vi "LVDemo1-Z.vi"() -> ()   [LabVIEW 2016]
uses:
  toupcam.dll
  toupcam_labview.dll
panel:
  out "x/y":dbl
  out "10^x":dbl
  out "连接的字符串":string
  out "路径":path
  in  "下降步长":i32=3
  in  "step":i64(ring) items=["1", "10", "100", "1000", "10000"]
  in  "停止":bool
  in  "开始拍图":bool
  in  "Temp 3":i32
  in  "Tint 3":i32
  in  "Expotime 3":u32
  in  "ExpoGain 3":u16
  in  "Still_Width 2":i32
  in  "Still_Height 2":i32
  in  "Tab":T1(tab)
  in  "Color Default":bool
  in  "Brightness":i32(slide) scale=-64.0..64.0
  in  "Contrast":i32(slide) scale=-100.0..100.0
  in  "Gamma":i32(slide) scale=20.0..180.0
  in  "Hue":i32(slide) scale=-180.0..180.0
  in  "Saturation":i32(slide) scale=0.0..255.0
  in  "AutoExpo":bool
  in  "ExpoDefault":bool
  in  "Expotime":u32(slide) scale=100.0..3600000000.0
  in  "ExpoGain":u16(slide) scale=100.0..5000.0
  in  "AutoWB":bool
  in  "WBDefault":bool
  in  "Tint":i32(slide) scale=200.0..2500.0
  in  "Temp":i32(slide) scale=2000.0..15000.0
  in  "Bin/Skip Mode":bool
  in  "Chrome/Mono":bool
  in  "HFlip":bool
  in  "VFlip":bool
  in  "Frame Speed":u8(slide) scale=0.0..2.0
  out "Video":T2(plugin-control)
  in  "Cap Still Image":bool
  in  "Still Image Resolution":u16(ring) items=["3840*2160", "1920*1080"]
  in  "Cap Live Image":bool
  in  "Stop":bool
  in  "Live Resolution":u16(ring) items=["3840*2160", "1920*1080"]
  in  "?":enum32{"选项卡 1"}(tab)
  in  "Expotime_def":u32
  in  "ExpoGain_def":u16
  in  "ExpoGain_Max":u16
  in  "ExpoGain_Min":u16
  in  "Height":i32
  in  "Width":i32
  in  "Expotime_Max":u32
  in  "Expotime_Min":u32
  in  "speed":u8
  in  "height2":i32
  in  "width2":i32
  in  "Mode":bool
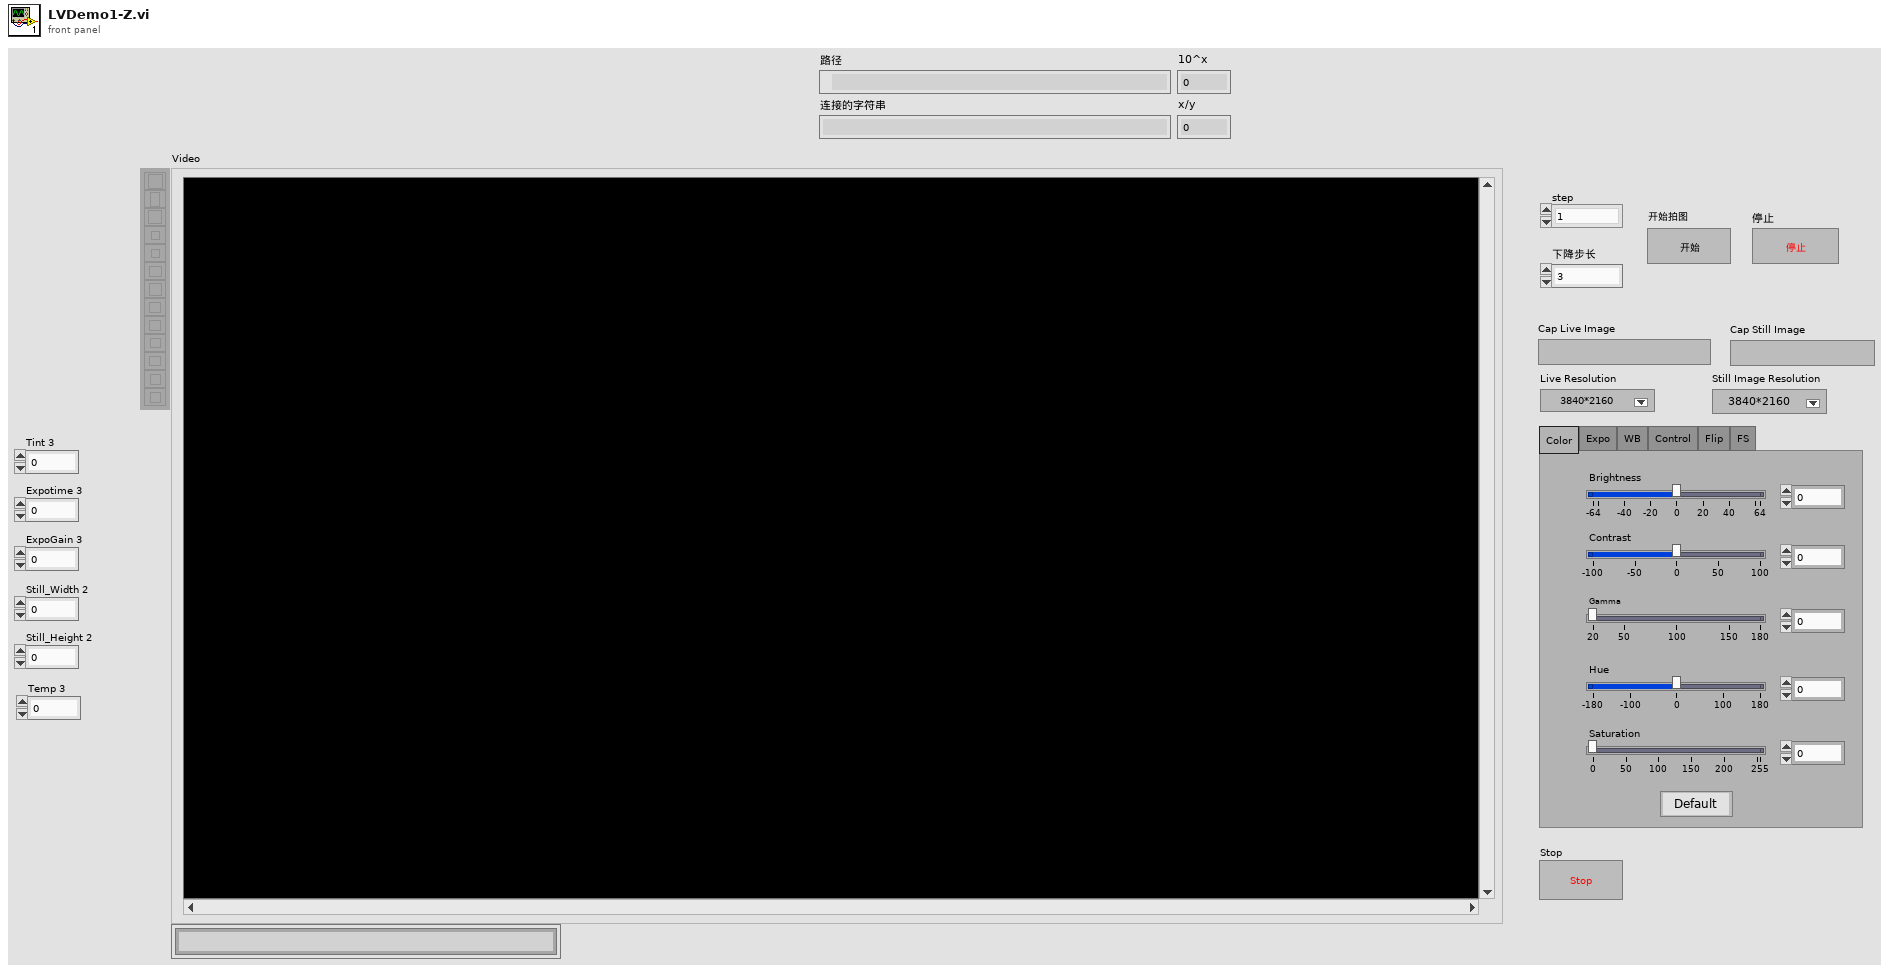
[diagram p1: front panel]
types:
  T1 = enum32{"Color", "Expo", "WB", "Control", "Flip", "FS"}
  T2 = typedef "IMAQ Image.ctl" = refnum<image>
  T3 = enum8{"Enabled", "Disabled", "Disabled and Grayed Out"}
  T4 = typedef "Image Type" = u32
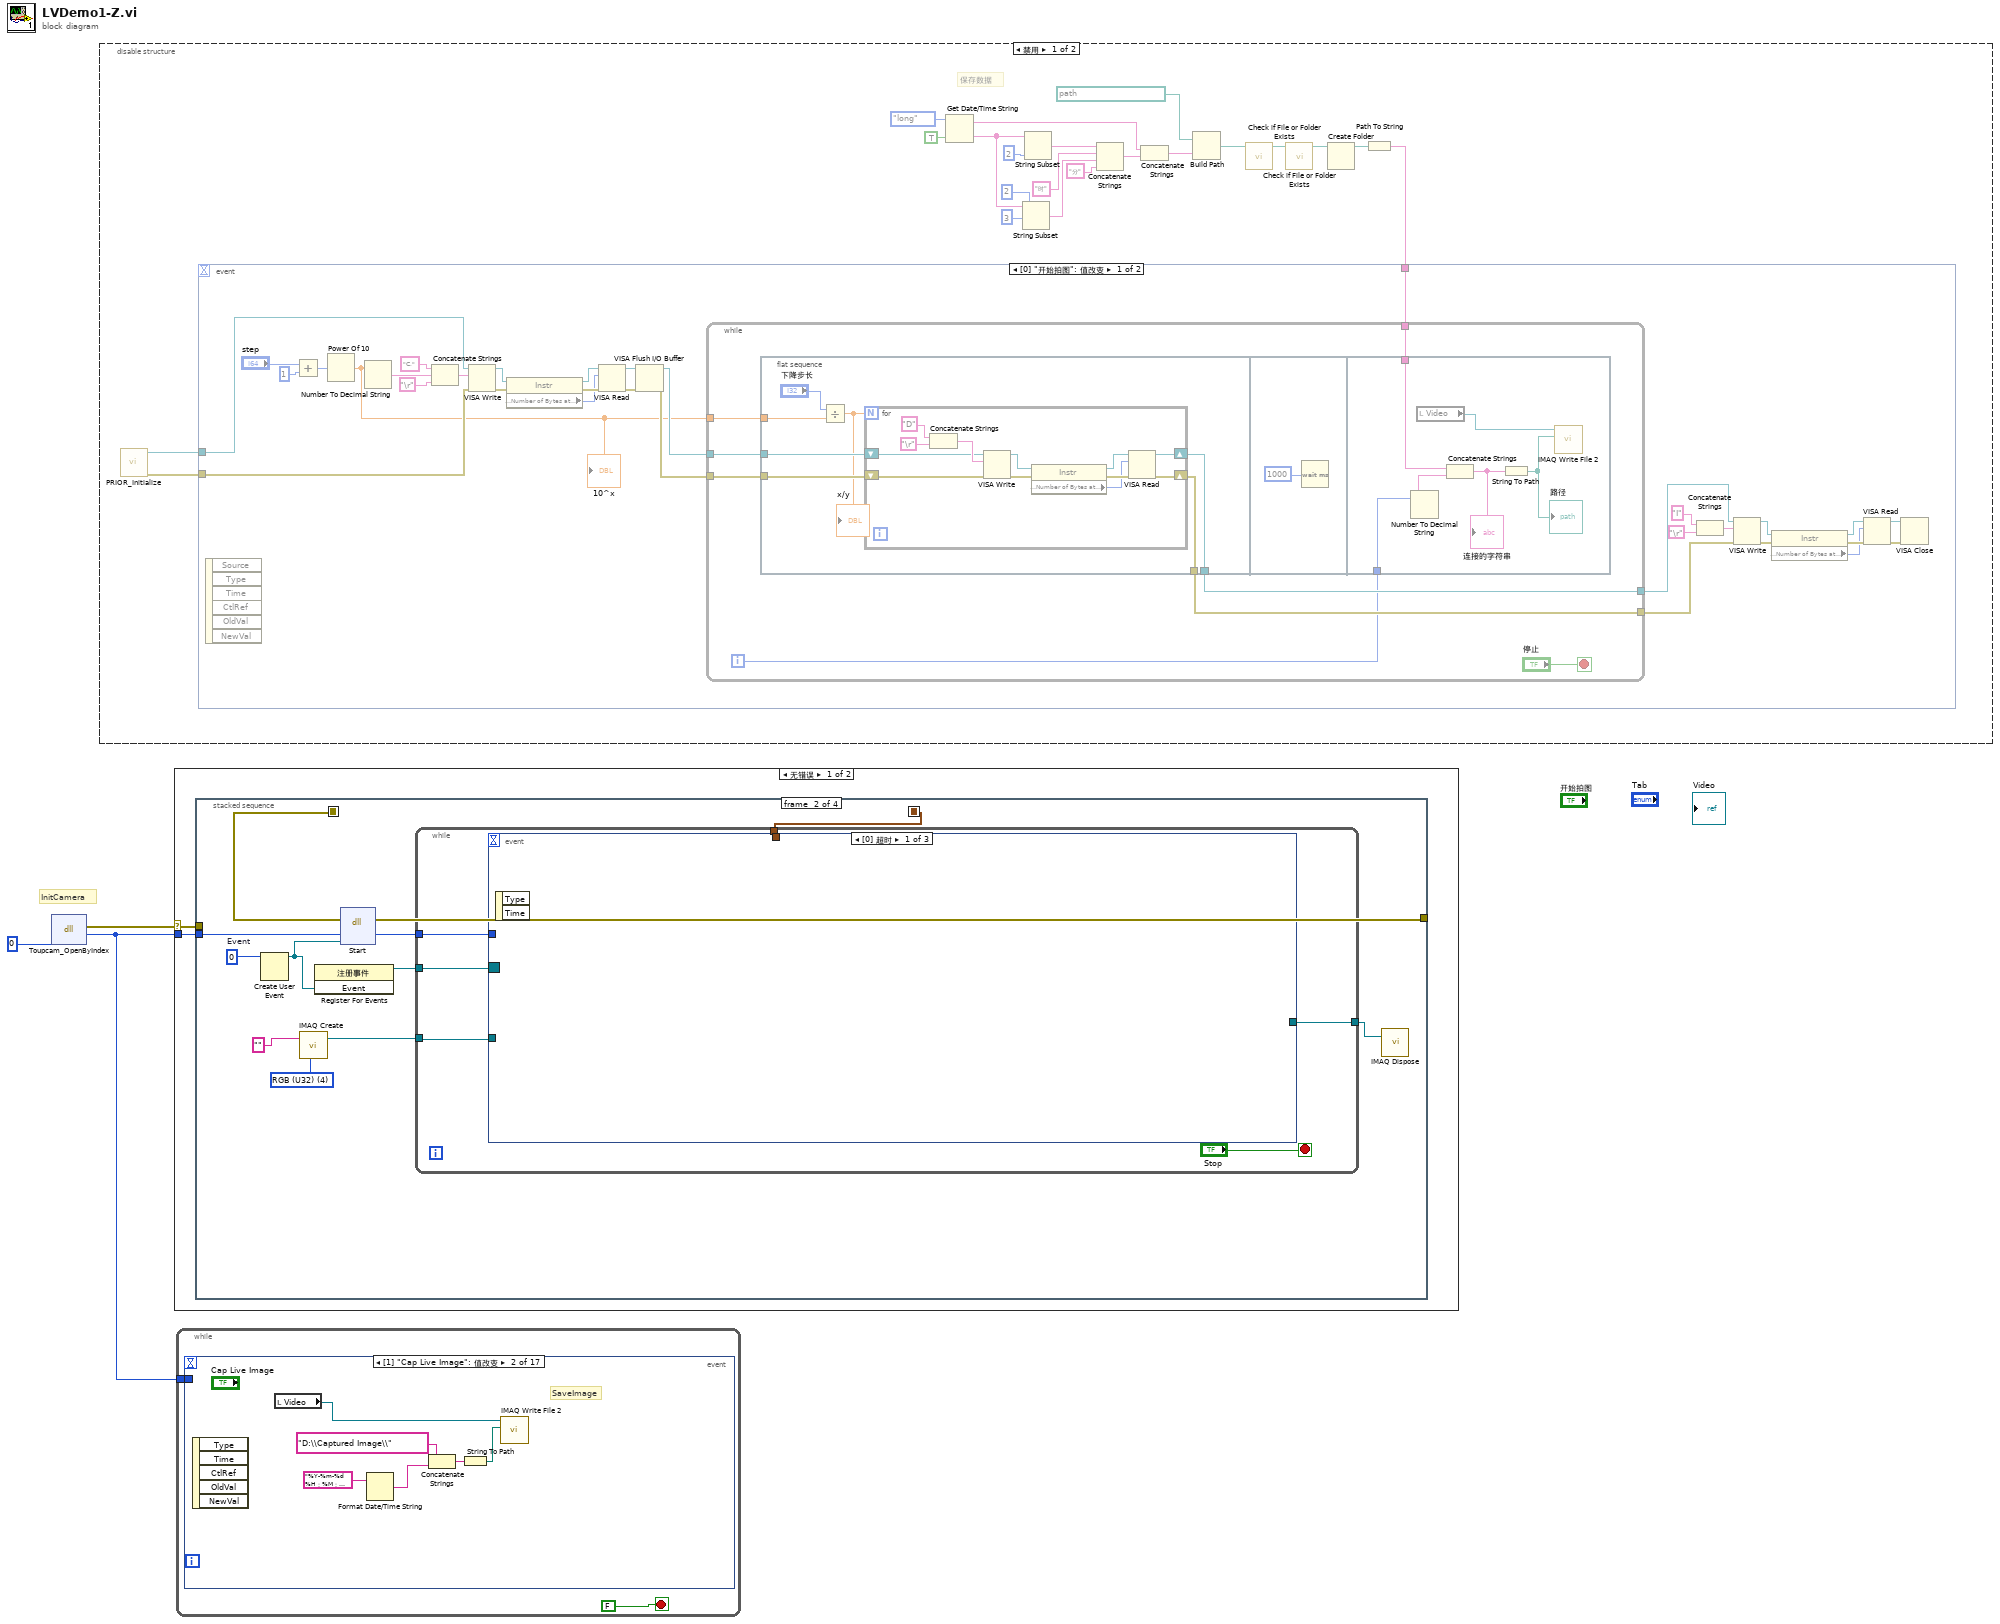
[diagram p0: block diagram]
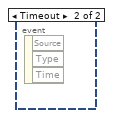
[diagram p2: hidden frame]
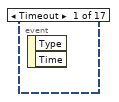
[diagram p4: hidden frame]
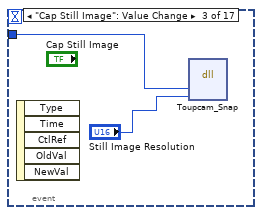
[diagram p5: hidden frame]
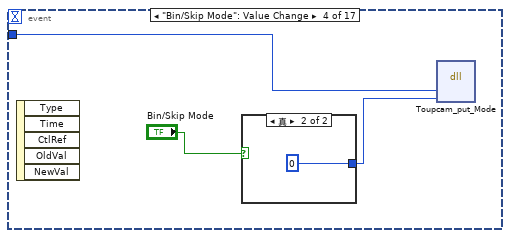
[diagram p6: hidden frame]
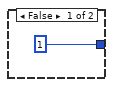
[diagram p7: hidden frame]
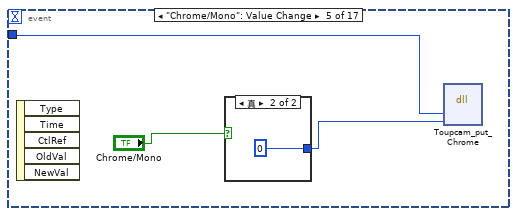
[diagram p8: hidden frame]
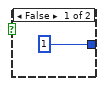
[diagram p9: hidden frame]
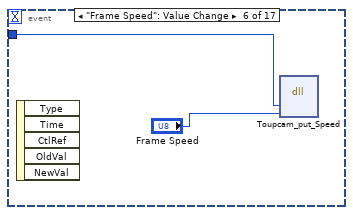
[diagram p10: hidden frame]
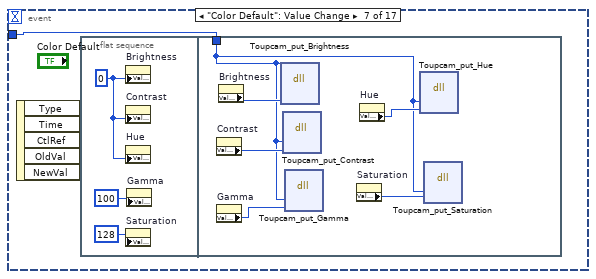
[diagram p11: hidden frame]
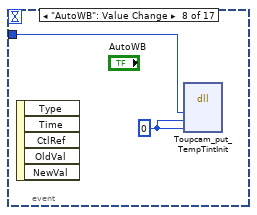
[diagram p12: hidden frame]
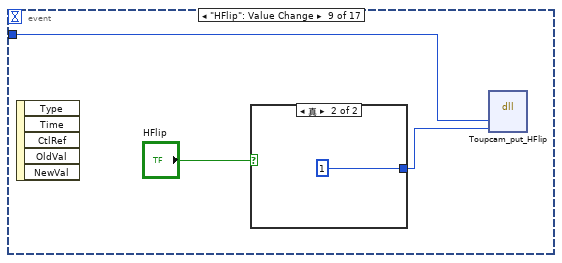
[diagram p13: hidden frame]
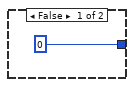
[diagram p14: hidden frame]
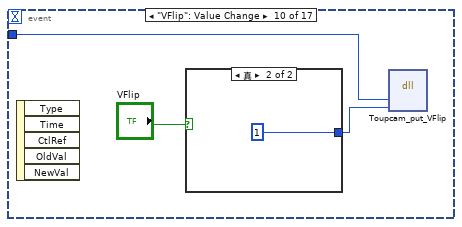
[diagram p15: hidden frame]
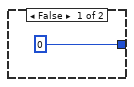
[diagram p16: hidden frame]
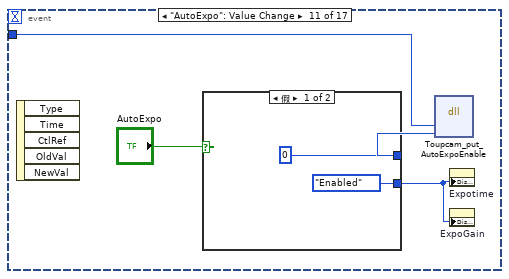
[diagram p17: hidden frame]
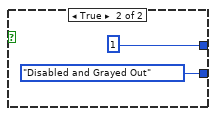
[diagram p18: hidden frame]
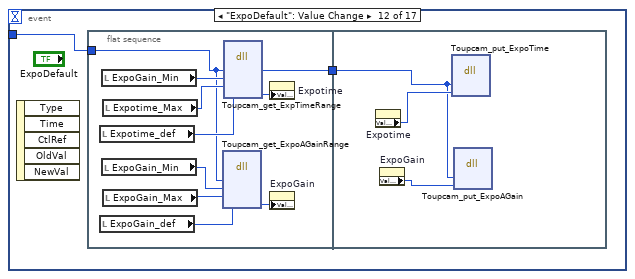
[diagram p19: hidden frame]
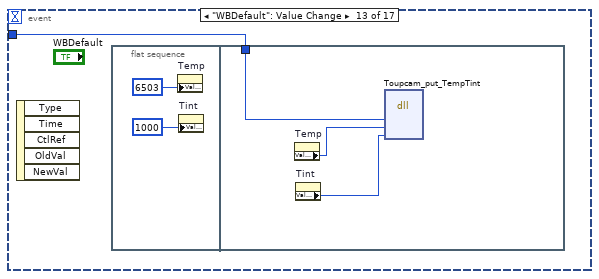
[diagram p20: hidden frame]
diagram:
  # "InitCamera"
  n1 = dll-call lib="PTH2=abs E膜片\t膜片钳程序自动拍图toupcam.dll" fn="Toupcam_OpenByIndex"("Index"=0) -> (error out=w3:errorcluster, "return type"=w2:i32)  [unwired: 4 in, 1 out]
  n2 = disable-structure shown="禁用" {
    frame Disabled {
      # "保存数据"
      n3 = call "PRIOR_Initialize.vi"() -> ("错误输出"=w23:errorcluster, "VISA资源名称输出"=w24:refnum<visa-resource-name>)  [unwired: 10 in]
      n4 = Get Date/Time String(date format (0)=enum16{"short", "long", "abbreviated"}."long" ("日期格式(0)"), want seconds? (F)=TRUE ("需要秒？(F)")) -> (date string=w22:string, time string=w13:string)  [unwired: 1 in]
      n5 = String Subset(string=w13, offset (0)=3 ("偏移量(0)"), length (rest)=2 ("长度（剩余）")) -> (substring=w17:string)
      n6 = String Subset(string=w13, length (rest)=2 ("长度（剩余）")) -> (substring=w19:string)  [unwired: 1 in]
      n7 = Concatenate Strings(w19, "时" ("字符串"), w17, "分" ("字符串")) -> (w18:string)
      n8 = Concatenate Strings(w22, w18) -> (w10:string)
      n9 = Build Path(base path=path "E:/膜片/图片和视频" ("文件路径（使用对话框）"), name or relative path=w10) -> (appended path=w4:path)
      n10 = call <vilib>:"Check if File or Folder Exists.vi"("path"=w4) -> ("dup path"=w6:path)  [unwired: 8 in, 2 out]
      n11 = call <vilib>:"Check if File or Folder Exists.vi"("path"=w6) -> ("dup path"=w5:path)  [unwired: 8 in, 2 out]
      n12 = Create Folder(path (use dialog)=w5) -> (created path=w8:path)  [unwired: 2 in, 2 out]
      n13 = Path To String(path=w8) -> (string=w7:string)
      n14 = event shown="[0] \"开始拍图\": 值改变" {
        selector: _ -> [_ _]
        dyn-events: _ -> [_ _]
        timeout: _ -> [_ _]
        tunnel: w24 -> [w56 _]
        tunnel: w23 -> [w55 _]
        tunnel: w7 -> [w25 _]
        event "开始拍图": Value Change {
          n15 = event-data() -> ()  [unwired: 1 in, 6 out]
          n16 = Add(x="step", y=i64 1) -> (x+y=w43:i64)
          n17 = Power Of 10(x=w43) -> (10^x=w26:dbl)
          "10^x" <- w26
          n18 = Number To Decimal String(number=w26) -> (decimal integer string=w45:string)  [unwired: 1 in]
          n19 = Concatenate Strings("C," ("写入缓冲区"), w45, "\r") -> (w47:string)
          n20 = VISA Write ("VISA写入")(VISA resource name=w56, write buffer=w47, error in (no error)=w55) -> (VISA resource name out=w51:refnum<visa-resource-name>, error out=w52:errorcluster)  [unwired: 1 out]
          n21 = property class="Instr"(reference=w51, error in=w52) -> (reference out=w50:refnum<visa-resource-name>, error out=w49:errorcluster, "Serial Settings:Number of Bytes at Serial Port"=w28:u32)
          n22 = VISA Read(VISA resource name=w50, byte count=w28, error in (no error)=w49) -> (VISA resource name out=w42:refnum<visa-resource-name>, error out=w41:errorcluster)  [unwired: 2 out]
          n23 = VISA Flush I/O Buffer(VISA resource name=w42, error in (no error)=w41) -> (VISA resource name out=w39:refnum<visa-resource-name>, error out=w40:errorcluster)  [unwired: 1 in]
          n24 = while {
            tunnel: [w64] -> w30
            tunnel: [w63] -> w29
            tunnel: w40 -> [w61]
            tunnel: w39 -> [w60]
            tunnel: w26 -> [w58]
            tunnel: w25 -> [w57]
            i -> [w62]
            stop <- "停止" stop-if-true
            n25 = flat-sequence {
              tunnel: [w71] -> w64
              tunnel: [w70] -> w63
              tunnel: w61 -> [w69]
              tunnel: w60 -> [w68]
              tunnel: w58 -> [w66]
              tunnel: w62 -> [w87]
              tunnel: w57 -> [w86]
              frame #0 {
                n26 = Divide(x="下降步长", y=w66) -> (x/y=w65:dbl)
                "x/y" <- w65
                n27 = for {
                  N: w65 -> [_]
                  shift-right: [w76] -> w70
                  shift-left: w69 -> [w75]
                  shift-right: [w77] -> w71
                  shift-left: w68 -> [w72]
                  n28 = Concatenate Strings("D" ("写入缓冲区"), "\r") -> (w83:string)
                  n29 = VISA Write ("VISA写入")(VISA resource name=w72, write buffer=w83, error in (no error)=w75) -> (VISA resource name out=w73:refnum<visa-resource-name>, error out=w78:errorcluster)  [unwired: 1 out]
                  n30 = property class="Instr"(reference=w73, error in=w78) -> (reference out=w79:refnum<visa-resource-name>, error out=w80:errorcluster, "Serial Settings:Number of Bytes at Serial Port"=w74:u32)
                  n31 = VISA Read(VISA resource name=w79, byte count=w74, error in (no error)=w80) -> (VISA resource name out=w77:refnum<visa-resource-name>, error out=w76:errorcluster)  [unwired: 2 out]
                }
              }
              frame #1 {
                n32 = Wait (ms)(milliseconds to wait=u32 1000 ("等待时间（毫秒）")) -> ()  [unwired: 1 out]
              }
              frame #2 {
                n33 = Number To Decimal String(number=w87) -> (decimal integer string=w85:string)  [unwired: 1 in]
                n34 = local read "Video"() -> (w90:T2)
                n35 = Concatenate Strings(w86, w85) -> (w89:string)
                "连接的字符串" <- w89
                n36 = String To Path(string=w89) -> (path=w88:path)
                "路径" <- w88
                n37 = call-poly "IMAQ Write File 2"("File Path"=w88, "Image"=w90) -> ()  [unwired: 8 in, 2 out]
              }
            }
          }
          n38 = Concatenate Strings("I" ("写入缓冲区"), "\r") -> (w31:string)
          n39 = VISA Write ("VISA写入")(VISA resource name=w30, write buffer=w31, error in (no error)=w29) -> (VISA resource name out=w37:refnum<visa-resource-name>, error out=w38:errorcluster)  [unwired: 1 out]
          n40 = property class="Instr"(reference=w37, error in=w38) -> (reference out=w36:refnum<visa-resource-name>, error out=w35:errorcluster, "Serial Settings:Number of Bytes at Serial Port"=w34:u32)
          n41 = VISA Read(VISA resource name=w36, byte count=w34, error in (no error)=w35) -> (VISA resource name out=w53:refnum<visa-resource-name>, error out=w54:errorcluster)  [unwired: 2 out]
          n42 = VISA Close(VISA resource name=w53, error in (no error)=w54) -> ()  [unwired: 1 out]
        }
        event Timeout {
          n43 = event-data() -> ()  [unwired: 1 in, 3 out]
        }
      }
    }
    frame Enabled {
    }
  }
  n44 = case shown="无错误" w3 {
    selector: w3 -> [w91 _]
    tunnel: w2 -> [w92 _]
    frame No Error {
      n45 = stacked-sequence {
        seq-local: [w113 _ _ _] -> [_ w159 _ _]
        seq-local: [w111 _ _ _] -> [_ w158 _ _]
        tunnel: w92 -> [w96 w156 w219 w222]
        tunnel: w91 -> [w111 _ _ w221]
        tunnel: [_ w157 _ _] -> _
        frame #0 {
          w93 = T3."Disabled and Grayed Out" ("禁用")
          w134 = 0
          # "SetSliderRange"
          # "SetCameraResolution"
          # "CameraResolution"
          # "SetSliderDefault"
          n46 = dll-call lib="PTH2=abs E膜片\t膜片钳程序自动拍图toupcam.dll" fn="Toupcam_put_AutoExpoEnable"("htoupcam"=w96, "bAutoExposure"=FALSE) -> ()  [unwired: 6 in, 2 out]
          n47 = dll-call lib="PTH2=abs E膜片\t膜片钳程序自动拍图toupcam.dll" fn="Toupcam_put_ExpoTime"("htoupcam"=w96, "Time"=5000) -> ()  [unwired: 6 in, 2 out]
          n48 = dll-call lib="PTH2=abs E膜片\t膜片钳程序自动拍图toupcam.dll" fn="Toupcam_get_ExpTimeRange"("htoupcam"=w96, "nMin"="Expotime_Min", "nMax"="Expotime_Max", "ndef"="Expotime_def") -> ("nMin"=w116:u32, "nMax"=w115:u32, "ndef"=w114:u32)  [unwired: 5 in, 2 out]
          n49 = dll-call lib="PTH2=abs E膜片\t膜片钳程序自动拍图toupcam.dll" fn="Toupcam_get_ExpoAGainRange"("htoupcam"=w96, "nmin"="ExpoGain_Min", "nmax"="ExpoGain_Max", "ndef"="ExpoGain_def") -> ("nmin"=w125:u16, "nmax"=w124:u16, "ndef"=w123:u16)  [unwired: 5 in, 2 out]
          n50 = property on="Expotime" class="Slide (strict)"("Scale.Minimum"=w116, "Scale.Maximum"=w115, "Value"=w114) -> ()  [unwired: 2 in, 2 out]
          n51 = property on="ExpoGain" class="Slide (严格)"("Scale.Minimum"=w125, "Scale.Maximum"=w124, "Value"=w123) -> ()  [unwired: 2 in, 2 out]
          n52 = dll-call lib="PTH2=abs E膜片\t膜片钳程序自动拍图toupcam.dll" fn="Toupcam_get_ResolutionNumber"("htoupcam"=w96) -> ("返回类型"=w102:u32, "htoupcam"=w101:i32)  [unwired: 3 in, 2 out]
          n53 = dll-call lib="PTH2=abs E膜片\t膜片钳程序自动拍图toupcam.dll" fn="Toupcam_get_Mode"("htoupcam"=w96, "bMode"="Mode") -> ("返回类型"=w95:i32)  [unwired: 5 in, 2 out]
          n54 = property on="Expotime" class="Slide (strict)"("DisabledEnum"=w93) -> ()  [unwired: 2 in, 2 out]
          n55 = property on="ExpoGain" class="Slide (strict)"("DisabledEnum"=w93) -> ()  [unwired: 2 in, 2 out]
          n56 = Equal To 0?(x=w95) -> (x = 0?=w94:bool)
          n57 = dll-call lib="PTH2=abs E膜片\t膜片钳程序自动拍图toupcam.dll" fn="Toupcam_get_MaxSpeed"("htoupcam"=w96) -> ("返回类型"=w106:u8)  [unwired: 4 in, 2 out]
          n58 = dll-call lib="PTH2=abs E膜片\t膜片钳程序自动拍图toupcam.dll" fn="Toupcam_get_Speed"("htoupcam"=w96, "speed"="speed") -> ("htoupcam"=w104:i32, "speed"=w107:u8)  [unwired: 4 in, 2 out]
          n59 = for {
            N: w102 -> [_]
            tunnel: w101 -> [w148]
            tunnel: [w139] -> w100 mode=indexing
            i -> [w140]
            # "Enum Res"
            n60 = dll-call lib="PTH2=abs E膜片\t膜片钳程序自动拍图toupcam.dll" fn="Toupcam_get_Resolution"("htoupcam"=w148, "ResNum"=w140, "pWidth"="width2", "pHeight"="height2") -> ("pWidth"=w142:i32, "pHeight"=w141:i32)  [unwired: 6 in, 2 out]
            n61 = Number To Decimal String(number=w142) -> (decimal integer string=w143:string)  [unwired: 1 in]
            n62 = Number To Decimal String(number=w141) -> (decimal integer string=w145:string)  [unwired: 1 in]
            n63 = Concatenate Strings(w143, "*", w145) -> (w139:string)
          }
          n64 = case shown="假" w94 {
            frame True {
              n65 = property on="Bin/Skip Mode" class="Bool (严格)"("DisabledEnum"=T3."Enabled" ("禁用")) -> ()  [unwired: 2 in, 2 out]
            }
            frame False {
              n66 = property on="Bin/Skip Mode" class="Bool (严格)"("DisabledEnum"=T3."Disabled and Grayed Out" ("禁用")) -> ()  [unwired: 2 in, 2 out]
            }
          }
          n67 = property on="Frame Speed" class="Slide (严格)"("Value"=w107, "Scale.Maximum"=w106, "Scale.Minimum"=0) -> ()  [unwired: 2 in, 2 out]
          n68 = dll-call lib="PTH2=abs E膜片\t膜片钳程序自动拍图toupcam.dll" fn="Toupcam_get_MonoMode"("htoupcam"=w104) -> ("返回类型"=w103:i32)  [unwired: 4 in, 2 out]
          n69 = case shown="0, 默认" w103 {
            frame 0, Default {
              w149 = T3."Disabled and Grayed Out" ("禁用")
              # "Mono"
              n70 = property on="Brightness" class="Slide (严格)"("DisabledEnum"=w149) -> ()  [unwired: 2 in, 2 out]
              n71 = property on="Hue" class="Slide (严格)"("DisabledEnum"=w149) -> ()  [unwired: 2 in, 2 out]
              n72 = property on="Contrast" class="Slide (严格)"("DisabledEnum"=w149) -> ()  [unwired: 2 in, 2 out]
              n73 = property on="Gamma" class="Slide (严格)"("DisabledEnum"=w149) -> ()  [unwired: 2 in, 2 out]
              n74 = property on="AutoWB" class="Bool"("DisabledEnum"=w149) -> ()  [unwired: 2 in, 2 out]
              n75 = property on="Temp" class="Slide (严格)"("DisabledEnum"=w149) -> ()  [unwired: 2 in, 2 out]
              n76 = property on="Tint" class="Slide (严格)"("DisabledEnum"=w149) -> ()  [unwired: 2 in, 2 out]
              n77 = property on="Saturation" class="Slide (严格)"("DisabledEnum"=w149) -> ()  [unwired: 2 in, 2 out]
              n78 = property on="WBDefault" class="Bool"("DisabledEnum"=w149) -> ()  [unwired: 2 in, 2 out]
              n79 = property on="Color Default" class="Bool"("DisabledEnum"=w149) -> ()  [unwired: 2 in, 2 out]
            }
            frame 1 {
              w150 = T3."Enabled" ("禁用")
              # "Mono"
              n80 = property on="Brightness" class="Slide (严格)"("DisabledEnum"=w150) -> ()  [unwired: 2 in, 2 out]
              n81 = property on="Hue" class="Slide (严格)"("DisabledEnum"=w150) -> ()  [unwired: 2 in, 2 out]
              n82 = property on="Contrast" class="Slide (严格)"("DisabledEnum"=w150) -> ()  [unwired: 2 in, 2 out]
              n83 = property on="Gamma" class="Slide (严格)"("DisabledEnum"=w150) -> ()  [unwired: 2 in, 2 out]
              n84 = property on="AutoWB" class="Bool"("DisabledEnum"=w150) -> ()  [unwired: 2 in, 2 out]
              n85 = property on="Temp" class="Slide (严格)"("DisabledEnum"=w150) -> ()  [unwired: 2 in, 2 out]
              n86 = property on="Tint" class="Slide (严格)"("DisabledEnum"=w150) -> ()  [unwired: 2 in, 2 out]
              n87 = property on="Saturation" class="Slide (严格)"("DisabledEnum"=w150) -> ()  [unwired: 2 in, 2 out]
              n88 = property on="WBDefault" class="Bool"("DisabledEnum"=w150) -> ()  [unwired: 2 in, 2 out]
              n89 = property on="Color Default" class="Bool"("DisabledEnum"=w150) -> ()  [unwired: 2 in, 2 out]
            }
          }
          n90 = dll-call lib="PTH2=abs E膜片\t膜片钳程序自动拍图toupcam.dll" fn="Toupcam_get_Resolution"("htoupcam"=w101, "ResNum"="Live Resolution", "pWidth"="Width", "pHeight"="Height") -> ("pWidth"=w126:i32, "pHeight"=w127:i32)  [unwired: 6 in, 2 out]
          n91 = dll-call lib="PTH2=abs E膜片\t膜片钳程序自动拍图toupcam.dll" fn="Toupcam_put_eSize"("htoupcam"=w101, "nResolutionIndex"="Live Resolution") -> ()  [unwired: 6 in, 2 out]
          n92 = property on="Live Resolution" class="Ring (严格)"("Strings []"=w100) -> ()  [unwired: 2 in, 2 out]
          n93 = property on="Still Image Resolution" class="Ring (严格)"("Strings []"=w100) -> ()  [unwired: 2 in, 2 out]
          n94 = Bundle("pWidth"=w126, "pHeight"=w127) -> (w113:cluster{"pWidth":i32, "pHeight":i32})  [unwired: 1 in]
          n95 = property on="Brightness" class="Slide (严格)"("Value"=w134) -> ()  [unwired: 2 in, 2 out]
          n96 = property on="Contrast" class="Slide (严格)"("Value"=w134) -> ()  [unwired: 2 in, 2 out]
          n97 = property on="Hue" class="Slide (严格)"("Value"=w134) -> ()  [unwired: 2 in, 2 out]
          n98 = property on="Gamma" class="Slide (严格)"("Value"=100) -> ()  [unwired: 2 in, 2 out]
          n99 = property on="Saturation" class="Slide (严格)"("Value"=128) -> ()  [unwired: 2 in, 2 out]
          n100 = property on="Temp" class="Slide (严格)"("Value"=6503) -> ()  [unwired: 2 in, 2 out]
          n101 = property on="Tint" class="Slide (严格)"("Value"=1000) -> ()  [unwired: 2 in, 2 out]
          n102 = property on="AutoExpo" class="Bool (严格)"("Value"=TRUE) -> ()  [unwired: 2 in, 2 out]
          n103 = property on="Bin/Skip Mode" class="Bool (严格)"("Value"=TRUE) -> ()  [unwired: 2 in, 2 out]
          n104 = property on="Chrome/Mono" class="Bool (严格)"("Value"=TRUE) -> ()  [unwired: 2 in, 2 out]
          n105 = property class="TabCtl (严格)"("Visible"=FALSE) -> ()  [unwired: 2 in, 2 out]
        }
        frame #1 {
          w155 = u32 0  # Event
          w160 = T4 4 items=["Grayscale (U8)", "Grayscale (I16)", "Grayscale (SGL)", "Complex (CSG)", "RGB (U32)", "HSL (U32)", "RGB (U64)", "Grayscale (U16)"] ("Image Type")
          n106 = Create User Event(user event datatype=w155) -> (user event=w154:refnum<user-event>)  [unwired: 1 in, 1 out]
          n107 = call "IMAQ Create"("Image Name"="", "Image Type"=w160) -> ("New Image"=w161:T2)  [unwired: 3 in, 1 out]
          n108 = register-events(w154) -> (reference out=w153:refnum<event-registration>)  [unwired: 2 in, 1 out]
          n109 = dll-call lib="PTH2Eabs E膜片\t膜片钳程序自动拍图toupcam_labview.dll" fn="Start"(error in=w158, "htoupcam"=w156, "rwer"=w154) -> (error out=w157:errorcluster, "htoupcam"=w152:i32)  [unwired: 4 in, 1 out]
          n110 = while {
            tunnel: w161 -> [w167]
            tunnel: w159 -> [w166]
            tunnel: w153 -> [w165]
            tunnel: w152 -> [w164]
            tunnel: [w163] -> w151
            stop <- "Stop" stop-if-true
            n111 = event shown="[0] 超时" {
              selector: w165 -> [_ _ _]
              dyn-events: _ -> [_ _ _]
              timeout: _ -> [_ _ _]
              tunnel: w167 -> [_ w173 w216]
              tunnel: w166 -> [_ w172 _]
              tunnel: w164 -> [_ w170 w218]
              tunnel: [_ w169 _] -> w163
              event Timeout {
                n112 = event-data() -> ()  [unwired: 1 in, 2 out]
              }
              event User Event {
                n113 = event-data() -> ("Event"=w171:u32)  [unwired: 1 in]
                n114 = case shown="2" w171 {
                  tunnel: w173 -> [w184 w192 _ _ _]
                  tunnel: w172 -> [w180 _ _ _ _]
                  tunnel: w170 -> [w176 w187 w206 w211 _]
                  tunnel: [w174 w186 _ _ _] -> w169
                  frame 4, Default {
                    # "ShowVideo"
                    n115 = Unbundle(w180) -> ("pWidth"=w178:i32, "pHeight"=w177:i32)
                    n116 = Multiply(x=w178, y=w177) -> (x*y=w182:i32)
                    n117 = Initialize Array(u32 0, w182) -> (w179:u32[])
                    n118 = dll-call lib="PTH2=abs E膜片\t膜片钳程序自动拍图toupcam.dll" fn="Toupcam_PullImage"("htoupcam"=w176, "pImageData"=w179, "bits"=32, "nWidth"=w178, "nHeight"=w177) -> ("pImageData"=w185:u32[])  [unwired: 8 in, 2 out]
                    n119 = Reshape Array(w185, w177, w178) -> (w183:u32[][])
                    n120 = call "IMAQ ArrayToColorImage"("Image Pixels (U32)"=w183, "Image"=w184) -> ("Image Out"=w174:T2)  [unwired: 3 in, 1 out]
                    n121 = local write "Video"(w174) -> ()
                  }
                  frame 5 {
                    # "Capture still Image"
                    n122 = property on="Still Image Resolution" class="Ring (严格)"() -> ("Value"=w188:u16)  [unwired: 2 in, 2 out]
                    n123 = dll-call lib="PTH2=abs E膜片\t膜片钳程序自动拍图toupcam.dll" fn="Toupcam_get_StillResolution"("htoupcam"=w187, "nIndex"=w188, "pWidth"="Still_Width 2", "pHeight"="Still_Height 2") -> ("htoupcam"=w204:i32, "pWidth"=w190:i32, "pHeight"=w191:i32)  [unwired: 5 in, 2 out]
                    n124 = Multiply(x=w190, y=w191) -> (x*y=w189:i32)
                    n125 = Initialize Array(u32 0, w189) -> (w203:u32[])
                    n126 = dll-call lib="PTH2=abs E膜片\t膜片钳程序自动拍图toupcam.dll" fn="Toupcam_PullStillImage"("htoupcam"=w204, "pImageData"=w203, "bits"=32, "pnWidth"=w190, "pnHeight"=w191) -> ("pImageData"=w201:u32[])  [unwired: 8 in, 2 out]
                    n127 = Reshape Array(w201, w191, w190) -> (w193:u32[][])
                    n128 = call "IMAQ ArrayToColorImage"("Image Pixels (U32)"=w193, "Image"=w192) -> ("Image Out"=w186:T2)  [unwired: 3 in, 1 out]
                    n129 = Format Date/Time String(time format string (%c)="%Y-%m-%d %H：%M：%S.bmp ") -> (date/time string=w197:string)  [unwired: 2 in]
                    n130 = Concatenate Strings("D:\\Captured Image\\", w197) -> (w194:string)
                    n131 = String To Path(string=w194) -> (path=w196:path)
                    n132 = call-poly "IMAQ Write File 2"("File Path"=w196, "Image"=w186) -> ()  [unwired: 8 in, 2 out]
                  }
                  frame 1 {
                    # "Auto Expo"
                    n133 = dll-call lib="PTH2=abs E膜片\t膜片钳程序自动拍图toupcam.dll" fn="Toupcam_get_ExpoAGain"("htoupcam"=w206, "ExpoGain"="ExpoGain 3") -> ("ExpoGain"=w207:u16)  [unwired: 5 in, 2 out]
                    n134 = dll-call lib="PTH2=abs E膜片\t膜片钳程序自动拍图toupcam.dll" fn="Toupcam_get_ExpoTime"("htoupcam"=w206, "Expotime"="Expotime 3") -> ("Expotime"=w208:u32)  [unwired: 5 in, 2 out]
                    n135 = property on="ExpoGain" class="Slide (严格)"("Value"=w207) -> ()  [unwired: 2 in, 2 out]
                    n136 = property on="Expotime" class="Slide (严格)"("Value"=w208) -> ()  [unwired: 2 in, 2 out]
                  }
                  frame 2 {
                    # "Auto WhiteBalance"
                    n137 = dll-call lib="PTH2=abs E膜片\t膜片钳程序自动拍图toupcam.dll" fn="Toupcam_get_TempTint"("htoupcam"=w211, "Temp"="Temp 3", "Tint"="Tint 3") -> ("Temp"=w213:i32, "Tint"=w212:i32)  [unwired: 5 in, 2 out]
                    n138 = property on="Tint" class="Slide (严格)"("Value"=w212) -> ()  [unwired: 2 in, 2 out]
                    n139 = property on="Temp" class="Slide (严格)"("Value"=w213) -> ()  [unwired: 2 in, 2 out]
                  }
                  frame 3 {
                  }
                }
              }
              event Application Instance Close {
                n140 = event-data() -> ()  [unwired: 1 in, 1 out]
                n141 = call "IMAQ Dispose"("Image"=w216) -> ()  [unwired: 5 in, 1 out]
                n142 = dll-call lib="PTH2=abs E膜片\t膜片钳程序自动拍图toupcam.dll" fn="Toupcam_Stop"("htoupcam"=w218) -> ("htoupcam"=w217:i32)  [unwired: 4 in, 2 out]
                n143 = dll-call lib="PTH2=abs E膜片\t膜片钳程序自动拍图toupcam.dll" fn="Toupcam_Close"("htoupcam"=w217) -> ()  [unwired: 5 in, 2 out]
              }
            }
          }
          n144 = call "IMAQ Dispose"("Image"=w151) -> ()  [unwired: 5 in, 1 out]
        }
        frame #2 {
          n145 = dll-call lib="PTH2=abs E膜片\t膜片钳程序自动拍图toupcam.dll" fn="Toupcam_Stop"("htoupcam"=w219) -> ()  [unwired: 5 in, 2 out]
        }
        frame #3 {
          n146 = dll-call lib="PTH2=abs E膜片\t膜片钳程序自动拍图toupcam.dll" fn="Toupcam_Close"(error in=w221, "htoupcam"=w222) -> ()  [unwired: 4 in, 2 out]
          n147 = Stop(stop? (T)=TRUE) -> ()
        }
      }
    }
    frame Error {
    }
  }
  n148 = while {
    tunnel: w2 -> [w223]
    stop <- FALSE ("停止 2") stop-if-true
    n149 = event shown="[1] \"Cap Live Image\": 值改变" {
      selector: _ -> [_ _ _ _ _ _ _ _ _ _ _ _ _ _ _ _ _]
      dyn-events: _ -> [_ _ _ _ _ _ _ _ _ _ _ _ _ _ _ _ _]
      timeout: _ -> [_ _ _ _ _ _ _ _ _ _ _ _ _ _ _ _ _]
      tunnel: w223 -> [_ _ w232 w235 w240 w243 w245 w256 w259 w264 w270 w276 w290 w297 w303 w305 w309]
      event Timeout {
        n150 = event-data() -> ()  [unwired: 1 in, 2 out]
      }
      event "Cap Live Image": Value Change {
        # "SaveImage"
        n151 = event-data() -> ()  [unwired: 1 in, 5 out]
        n152 = local read "Video"() -> (w225:T2)
        n153 = Format Date/Time String(time format string (%c)="%Y-%m-%d %H：%M：%S.bmp ") -> (date/time string=w229:string)  [unwired: 2 in]
        n154 = Concatenate Strings("D:\\Captured Image\\", w229) -> (w226:string)
        n155 = String To Path(string=w226) -> (path=w228:path)
        n156 = call-poly "IMAQ Write File 2"("File Path"=w228, "Image"=w225) -> ()  [unwired: 8 in, 2 out]
      }
      event "Cap Still Image": Value Change {
        n157 = event-data() -> ()  [unwired: 1 in, 5 out]
        n158 = dll-call lib="PTH2=abs E膜片\t膜片钳程序自动拍图toupcam.dll" fn="Toupcam_Snap"("htoupcam"=w232, "ResIndex"="Still Image Resolution") -> ()  [unwired: 6 in, 2 out]
      }
      event "Bin/Skip Mode": Value Change {
        n159 = event-data() -> ()  [unwired: 1 in, 5 out]
        n160 = case shown="真" "Bin/Skip Mode" {
          tunnel: [1 0] -> w233
          frame False {
          }
          frame True {
          }
        }
        n161 = dll-call lib="PTH2=abs E膜片\t膜片钳程序自动拍图toupcam.dll" fn="Toupcam_put_Mode"("htoupcam"=w235, "mode"=w233) -> ()  [unwired: 6 in, 2 out]
      }
      event "Chrome/Mono": Value Change {
        n162 = event-data() -> ()  [unwired: 1 in, 5 out]
        n163 = case shown="真" "Chrome/Mono" {
          tunnel: [1 0] -> w238
          frame False {
          }
          frame True {
          }
        }
        n164 = dll-call lib="PTH2=abs E膜片\t膜片钳程序自动拍图toupcam.dll" fn="Toupcam_put_Chrome"("htoupcam"=w240, "chrome"=w238) -> ()  [unwired: 6 in, 2 out]
      }
      event "Frame Speed": Value Change {
        n165 = event-data() -> ()  [unwired: 1 in, 5 out]
        n166 = dll-call lib="PTH2=abs E膜片\t膜片钳程序自动拍图toupcam.dll" fn="Toupcam_put_Speed"("htoupcam"=w243, "Speed"="Frame Speed") -> ()  [unwired: 6 in, 2 out]
      }
      event "Color Default": Value Change {
        n167 = event-data() -> ()  [unwired: 1 in, 5 out]
        n168 = flat-sequence {
          tunnel: w245 -> [w249]
          frame #0 {
            w248 = 0
            n169 = property on="Brightness" class="Slide (严格)"("Value"=w248) -> ()  [unwired: 2 in, 2 out]
            n170 = property on="Contrast" class="Slide (严格)"("Value"=w248) -> ()  [unwired: 2 in, 2 out]
            n171 = property on="Hue" class="Slide (严格)"("Value"=w248) -> ()  [unwired: 2 in, 2 out]
            n172 = property on="Saturation" class="Slide (严格)"("Value"=128) -> ()  [unwired: 2 in, 2 out]
            n173 = property on="Gamma" class="Slide (严格)"("Value"=100) -> ()  [unwired: 2 in, 2 out]
          }
          frame #1 {
            n174 = property on="Contrast" class="Slide (严格)"() -> ("Value"=w253:i32)  [unwired: 2 in, 2 out]
            n175 = property on="Gamma" class="Slide (严格)"() -> ("Value"=w252:i32)  [unwired: 2 in, 2 out]
            n176 = property on="Brightness" class="Slide (严格)"() -> ("Value"=w254:i32)  [unwired: 2 in, 2 out]
            n177 = dll-call lib="PTH2=abs E膜片\t膜片钳程序自动拍图toupcam.dll" fn="Toupcam_put_Brightness"("htoupcam"=w249, "Brightness"=w254) -> ()  [unwired: 6 in, 2 out]
            n178 = dll-call lib="PTH2=abs E膜片\t膜片钳程序自动拍图toupcam.dll" fn="Toupcam_put_Contrast"("htoupcam"=w249, "Contrast"=w253) -> ()  [unwired: 6 in, 2 out]
            n179 = dll-call lib="PTH2=abs E膜片\t膜片钳程序自动拍图toupcam.dll" fn="Toupcam_put_Gamma"("htoupcam"=w249, "Gamma"=w252) -> ()  [unwired: 6 in, 2 out]
            n180 = property on="Saturation" class="Slide (严格)"() -> ("Value"=w250:i32)  [unwired: 2 in, 2 out]
            n181 = property on="Hue" class="Slide (严格)"() -> ("Value"=w251:i32)  [unwired: 2 in, 2 out]
            n182 = dll-call lib="PTH2=abs E膜片\t膜片钳程序自动拍图toupcam.dll" fn="Toupcam_put_Hue"("htoupcam"=w249, "Hue"=w251) -> ()  [unwired: 6 in, 2 out]
            n183 = dll-call lib="PTH2=abs E膜片\t膜片钳程序自动拍图toupcam.dll" fn="Toupcam_put_Saturation"("htoupcam"=w249, "Saturation"=w250) -> ()  [unwired: 6 in, 2 out]
          }
        }
      }
      event "AutoWB": Value Change {
        w255 = 0
        n184 = event-data() -> ()  [unwired: 1 in, 5 out]
        n185 = dll-call lib="PTH2=abs E膜片\t膜片钳程序自动拍图toupcam.dll" fn="Toupcam_put_TempTintInit"("htoupcam"=w256, "fnTTProc"=w255, "pTTCtx"=w255) -> ()  [unwired: 7 in, 2 out]
      }
      event "HFlip": Value Change {
        n186 = event-data() -> ()  [unwired: 1 in, 5 out]
        n187 = case shown="真" "HFlip" {
          tunnel: [0 1] -> w257
          frame False {
          }
          frame True {
          }
        }
        n188 = dll-call lib="PTH2=abs E膜片\t膜片钳程序自动拍图toupcam.dll" fn="Toupcam_put_HFlip"("htoupcam"=w259, "bHFlip"=w257) -> ()  [unwired: 6 in, 2 out]
      }
      event "VFlip": Value Change {
        n189 = event-data() -> ()  [unwired: 1 in, 5 out]
        n190 = case shown="真" "VFlip" {
          tunnel: [0 1] -> w262
          frame False {
          }
          frame True {
          }
        }
        n191 = dll-call lib="PTH2=abs E膜片\t膜片钳程序自动拍图toupcam.dll" fn="Toupcam_put_VFlip"("htoupcam"=w264, "bVFlip"=w262) -> ()  [unwired: 6 in, 2 out]
      }
      event "AutoExpo": Value Change {
        n192 = event-data() -> ()  [unwired: 1 in, 5 out]
        n193 = case shown="假" "AutoExpo" {
          tunnel: [0 1] -> w267
          tunnel: [T3."Enabled" ("禁用") T3."Disabled and Grayed Out" ("禁用")] -> w268
          frame False {
          }
          frame True {
          }
        }
        n194 = dll-call lib="PTH2=abs E膜片\t膜片钳程序自动拍图toupcam.dll" fn="Toupcam_put_AutoExpoEnable"("HToupcam"=w270, "bAutoExposure"=w267) -> ()  [unwired: 6 in, 2 out]
        n195 = property on="Expotime" class="Slide (严格)"("DisabledEnum"=w268) -> ()  [unwired: 2 in, 2 out]
        n196 = property on="ExpoGain" class="Slide (严格)"("DisabledEnum"=w268) -> ()  [unwired: 2 in, 2 out]
      }
      event "ExpoDefault": Value Change {
        n197 = event-data() -> ()  [unwired: 1 in, 5 out]
        n198 = flat-sequence {
          tunnel: w276 -> [w278]
          tunnel: [w277] -> w275
          tunnel: w275 -> [w287]
          frame #0 {
            n199 = local read "Expotime_def"() -> (w284:u32)
            n200 = local read "ExpoGain_def"() -> (w280:u16)
            n201 = local read "ExpoGain_Min"() -> (w286:u16)
            n202 = local read "ExpoGain_Min"() -> (w282:u16)
            n203 = local read "Expotime_Max"() -> (w285:u32)
            n204 = local read "ExpoGain_Max"() -> (w281:u16)
            n205 = dll-call lib="PTH2=abs E膜片\t膜片钳程序自动拍图toupcam.dll" fn="Toupcam_get_ExpoAGainRange"("htoupcam"=w278, "min"=w282, "max"=w281, "def"=w280) -> ("def"=w283:u16)  [unwired: 7 in, 2 out]
            n206 = dll-call lib="PTH2=abs E膜片\t膜片钳程序自动拍图toupcam.dll" fn="Toupcam_get_ExpTimeRange"("htoupcam"=w278, "Min"=w286, "Max"=w285, "def"=w284) -> ("htoupcam"=w277:i32, "def"=w279:u32)  [unwired: 6 in, 2 out]
            n207 = property on="Expotime" class="Slide (严格)"("Value"=w279) -> ()  [unwired: 2 in, 2 out]
            n208 = property on="ExpoGain" class="Slide (严格)"("Value"=w283) -> ()  [unwired: 2 in, 2 out]
          }
          frame #1 {
            n209 = property on="Expotime" class="Slide (严格)"() -> ("Value"=w289:u32)  [unwired: 2 in, 2 out]
            n210 = property on="ExpoGain" class="Slide (严格)"() -> ("Value"=w288:u16)  [unwired: 2 in, 2 out]
            n211 = dll-call lib="PTH2=abs E膜片\t膜片钳程序自动拍图toupcam.dll" fn="Toupcam_put_ExpoTime"("htoupcam"=w287, "Expotime"=w289) -> ()  [unwired: 6 in, 2 out]
            n212 = dll-call lib="PTH2=abs E膜片\t膜片钳程序自动拍图toupcam.dll" fn="Toupcam_put_ExpoAGain"("htoupcam"=w287, "ExpoGain"=w288) -> ()  [unwired: 6 in, 2 out]
          }
        }
      }
      event "WBDefault": Value Change {
        n213 = event-data() -> ()  [unwired: 1 in, 5 out]
        n214 = flat-sequence {
          tunnel: w290 -> [w295]
          frame #0 {
            n215 = property on="Temp" class="Slide (严格)"("Value"=6503) -> ()  [unwired: 2 in, 2 out]
            n216 = property on="Tint" class="Slide (严格)"("Value"=1000) -> ()  [unwired: 2 in, 2 out]
          }
          frame #1 {
            n217 = property on="Temp" class="Slide (严格)"() -> ("Value"=w294:i32)  [unwired: 2 in, 2 out]
            n218 = property on="Tint" class="Slide (严格)"() -> ("Value"=w293:i32)  [unwired: 2 in, 2 out]
            n219 = dll-call lib="PTH2=abs E膜片\t膜片钳程序自动拍图toupcam.dll" fn="Toupcam_put_TempTint"("htoupcam"=w295, "Temp"=w294, "Tint"=w293) -> ()  [unwired: 7 in, 2 out]
          }
        }
      }
      event "Brightness", "Contrast", "Gamma", "Hue", "Saturation": Value Change {
        n220 = event-data() -> ()  [unwired: 1 in, 5 out]
        n221 = dll-call lib="PTH2=abs E膜片\t膜片钳程序自动拍图toupcam.dll" fn="Toupcam_put_Brightness"("htoupcam"=w297, "Brightness"="Brightness") -> ("htoupcam"=w296:i32)  [unwired: 5 in, 2 out]
        n222 = dll-call lib="PTH2=abs E膜片\t膜片钳程序自动拍图toupcam.dll" fn="Toupcam_put_Contrast"("htoupcam"=w297, "Contrast"="Contrast") -> ()  [unwired: 6 in, 2 out]
        n223 = dll-call lib="PTH2=abs E膜片\t膜片钳程序自动拍图toupcam.dll" fn="Toupcam_put_Gamma"("htoupcam"=w297, "Gamma"="Gamma") -> ()  [unwired: 6 in, 2 out]
        n224 = dll-call lib="PTH2=abs E膜片\t膜片钳程序自动拍图toupcam.dll" fn="Toupcam_put_Hue"("htoupcam"=w296, "Hue"="Hue") -> ()  [unwired: 6 in, 2 out]
        n225 = dll-call lib="PTH2=abs E膜片\t膜片钳程序自动拍图toupcam.dll" fn="Toupcam_put_Saturation"("htoupcam"=w296, "Saturation"="Saturation") -> ()  [unwired: 6 in, 2 out]
      }
      event "Expotime": Value Change {
        n226 = event-data() -> ()  [unwired: 1 in, 5 out]
        n227 = dll-call lib="PTH2=abs E膜片\t膜片钳程序自动拍图toupcam.dll" fn="Toupcam_put_ExpoTime"("htoupcam"=w303, "Expotime"="Expotime") -> ()  [unwired: 6 in, 2 out]
      }
      event "ExpoGain": Value Change {
        n228 = event-data() -> ()  [unwired: 1 in, 5 out]
        n229 = dll-call lib="PTH2=abs E膜片\t膜片钳程序自动拍图toupcam.dll" fn="Toupcam_put_ExpoAGain"("htoupcam"=w305, "ExpoGain"="ExpoGain") -> ()  [unwired: 6 in, 2 out]
      }
      event "Temp", "Tint": Value Change {
        n230 = event-data() -> ()  [unwired: 1 in, 5 out]
        n231 = dll-call lib="PTH2=abs E膜片\t膜片钳程序自动拍图toupcam.dll" fn="Toupcam_put_TempTint"("htoupcam"=w309, "Temp"="Temp", "Tint"="Tint") -> ()  [unwired: 7 in, 2 out]
      }
    }
  }
